vi "ExSpectGetSlitInfoDouble.vi"() -> ()   [LabVIEW 2010]
panel:
  out "Speed":dbl format="%.2f"
  out "Position":dbl format="%.2f"
  in  "Slit Number":i16=1 min=1 max=8 step=1
  out "error out":errorcluster
  in  "error in (no error)":errorcluster
  # "ExSpectGetSlitInfoDouble.vi\n(Normal Spectrograph via USB/COM port)\nThis VI will read the current position and speed of the selected slit."
  # "NOTES:\nA properly configured spectometer .ini must be present in the LabVIEW folder for spectrograph operation.\n\nConsult the Toolkit documentation for more information on how to configure this file."
  # "um"
  # "Master\n 1 = Front Entrance\n 2 = Side Entrance\n 3 = Front Exit\n 4 = Side Exit\n         Slave\n 5 = Front Entrance\n 6 = Side Entrance\n 7 = Front Exit\n 8 = Side Exit"
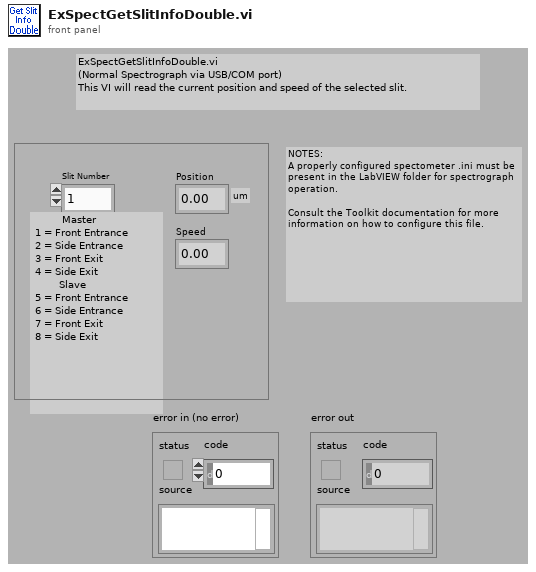
[diagram p1: front panel]
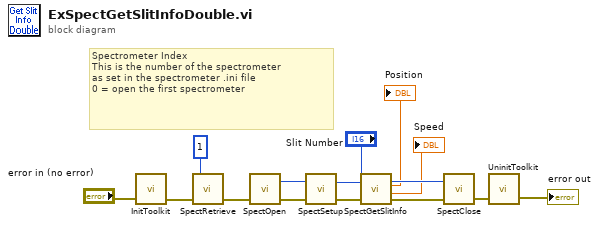
[diagram p0: block diagram]
diagram:
  # "Spectrometer Index\nThis is the number of the spectrometer\nas set in the spectrometer .ini file\n0 = open the first spectrometer"
  n1 = call <userlib>:"InitToolkit.vi"("error in"="error in (no error)") -> ("error out"=w2:errorcluster)
  n2 = call <userlib>:"SpectRetrieve.vi"("error in"=w2, "Index"=1) -> ("error out"=w4:errorcluster)  [unwired: 1 out]
  n3 = call <userlib>:"SpectOpen.vi"("error in"=w4) -> ("error out"=w14:errorcluster, "Spectrometer Handle"=w10:u32)  [unwired: 2 in]
  n4 = call <userlib>:"SpectSetup.vi"("error in"=w14, "Spectrometer Handle"=w10) -> ("error out"=w13:errorcluster, "Spectrometer Handle"=w9:u32)
  n5 = call <userlib>:"SpectGetSlitInfo.vi"("Spectrometer Handle"=w9, "Slit"="Slit Number", "error in"=w13) -> ("Spectrometer Handle"=w8:u32, "Position"=→"Position":dbl, "Speed"=→"Speed":dbl, "error out"=w12:errorcluster)
  n6 = call <userlib>:"SpectClose.vi"("error in"=w12, "Spectrometer Handle"=w8) -> ("error out"=w11:errorcluster)
  n7 = call <userlib>:"UninitToolkit.vi"("error in"=w11) -> ("error out"=→"error out":errorcluster)
